vi "Make Slow Read Mode File.vi"(8 "error in (no error)":errorcluster, 11 "Setup File in":refnum<class "Setup File.lvclass">) -> (0 "error out":errorcluster, 3 "Setup File out":refnum<class "Setup File.lvclass">)   [LabVIEW 2018, in "Setup File.lvclass"]
uses:
  Setup File.lvclass
  Setup File.lvclass/Setup File.ctl
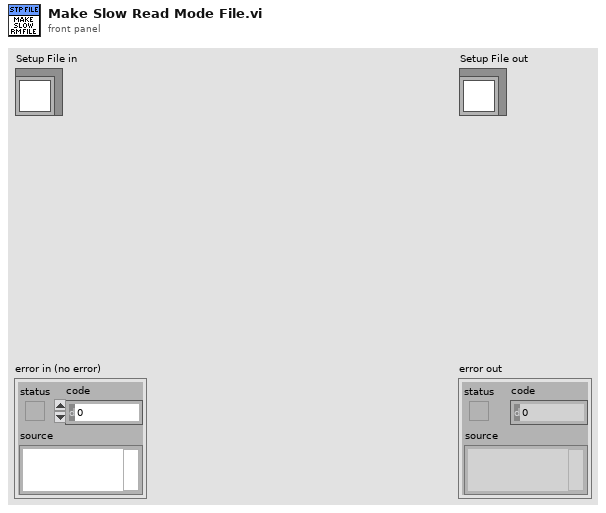
[diagram p1: front panel]
types:
  T1 = enum16{"open", "replace", "create", "open or create", "replace or create", "replace or create with confirmation"}
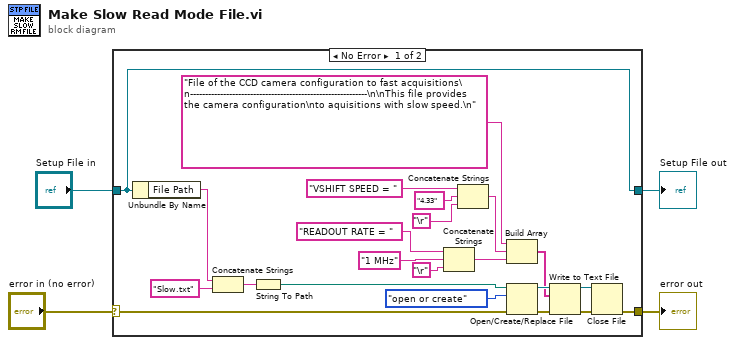
[diagram p0: block diagram]
diagram:
  n1 = case shown="No Error" "error in (no error)" {
    selector: "error in (no error)" -> [w26 w28]
    tunnel: [w23 w28] -> w2
    tunnel: [w20 w27] -> w3
    tunnel: "Setup File in" -> [w20 w27]
    frame No Error {
      n2 = Unbundle By Name(w20) -> ("File Path"=w19:string)
      n3 = Concatenate Strings(w19, "Slow.txt") -> (w18:string)
      n4 = String To Path(string=w18) -> (path=w17:path)
      n5 = Concatenate Strings("READOUT RATE = ", "1 MHz", "\r") -> (w11:string)
      n6 = Concatenate Strings("VSHIFT SPEED = ", "4.33", "\r") -> (w12:string)
      n7 = Build Array("File of the CCD camera configuration to fast acquisitions\n-----------------------------------------------------------\n\nThis file provides the camera configuration\nto aquisitions with slow speed.\n" ("string"), w12, w11) -> (w10:string[])
      n8 = Open/Create/Replace File(file path (use dialog)=w17, error in=w26, operation (0:open)=T1."open or create") -> (refnum out=w22:refnum<file>, error out=w25:errorcluster)  [unwired: 3 in, 1 out]
      n9 = Write to Text File(file (use dialog)=w22, text=w10, error in=w25) -> (refnum out=w21:refnum<file>, error out=w24:errorcluster)  [unwired: 1 in, 1 out]
      n10 = Close File(refnum=w21, error in=w24) -> (error out=w23:errorcluster)  [unwired: 1 out]
    }
    frame Error {
    }
  }
  "error out" <- w2
  "Setup File out" <- w3
